vi "raster sequence build.vi"() -> ()   [LabVIEW 2017]
uses:
  Classes/Sequence/SequenceSubvis/TestStep-StepType.ctl
  Classes/Sequence/SequenceSubvis/TestStepTypes.ctl
  Classes/Sequence/SequenceSubvis/RF Direction.ctl
  Classes/Sequence/SequenceSubvis/PolarizationSelect.ctl
  Classes/aparCfg/rasterConfig.ctl
  Classes/VXMCfg/VXMCfg.lvclass
  Classes/aparCfg/aparCfg.lvclass
panel:
  out "size(s)":i32
  out "Total points":dbl
  out "Raster Sequence":T1[](array[typedef])
  in  "Polarization":enum16{"Vertical", "Horizontal", "Both"}(ring)=enum."Both"
  in  "RF In/Out":T3
  out "apar properties.RasterDef":T5={"Nyquist, mm"=28.0, "Window, cm"=42.0}
  in  "Cfg File path":path=path "C:/Users/Public/Documents/UCAR/APAR Board Test/SupportFiles/aparConfig.ini"
  in  "Motion64.ini path":path=path "C:/Users/Public/Documents/UCAR/APAR Board Test/SupportFiles/Motion64.ini"
  out "TestZT":cluster{"Z mm":dbl, "Horizontal T deg":dbl}={"Z mm"=0.0, "Horizontal T deg"=1.0}
  out "TestSequence for P&M":T1[](array[typedef])=[{"StepType"=enum."Motion", "RF In/Out"=enum."Tx - RF In", "Module/Raster"=0, "Polarization"=enum."Vertical", "PhaseShift deg"=[], "Attenuation dB"=[], "Position"={"X mm"=204.374756, "Y mm"=144.119598, "Z mm"=0.0, "T deg"=-89.0}, "Patch RF In/Out"=TRUE}, {"StepType"=enum."SweepTest", "RF In/Out"=enum."Tx - RF In", "Module/Raster"=0, "Polarization"=enum."Vertical", "PhaseShift deg"=[0.0, 5.625, 11.25], "Attenuation dB"=[0.0, 0.5], "Position"={"X mm"=0.0, "Y mm"=0.0, "Z mm"=0.0, "T deg"=0.0}, "Patch RF In/Out"=FALSE}, {"StepType"=enum."Motion", "RF In/Out"=enum."Tx - RF In", "Module/Raster"=0, "Polarization"=enum."Horizontal", "PhaseShift deg"=[], "Attenuation dB"=[], "Position"={"X mm"=204.374756, "Y mm"=144.119598, "Z mm"=0.0, "T deg"=1.0}, "Patch RF In/Out"=FALSE}, {"StepType"=enum."SweepTest", "RF In/Out"=enum."Tx - RF In", "Module/Raster"=0, "Polarization"=enum."Horizontal", "PhaseShift deg"=[0.0, 5.625, 11.25], "Attenuation dB"=[0.0, 0.5], "Position"={"X mm"=0.0, "Y mm"=0.0, "Z mm"=0.0, "T deg"=0.0}, "Patch RF In/Out"=FALSE}, {"StepType"=enum."Motion", "RF In/Out"=enum."Tx - RF In", "Module/Raster"=4, "Polarization"=enum."Vertical", "PhaseShift deg"=[], "Attenuation dB"=[], "Position"={"X mm"=315.230015, "Y mm"=144.76588, "Z mm"=0.0, "T deg"=-89.0}, "Patch RF In/Out"=FALSE}, {"StepType"=enum."SweepTest", "RF In/Out"=enum."Tx - RF In", "Module/Raster"=4, "Polarization"=enum."Vertical", "PhaseShift deg"=[0.0, 5.625, 11.25], "Attenuation dB"=[0.5], "Position"={"X mm"=0.0, "Y mm"=0.0, "Z mm"=0.0, "T deg"=0.0}, "Patch RF In/Out"=FALSE}, {"StepType"=enum."Motion", "RF In/Out"=enum."Tx - RF In", "Module/Raster"=4, "Polarization"=enum."Horizontal", "PhaseShift deg"=[], "Attenuation dB"=[], "Position"={"X mm"=315.230015, "Y mm"=144.76588, "Z mm"=0.0, "T deg"=1.0}, "Patch RF In/Out"=FALSE}, {"StepType"=enum."SweepTest", "RF In/Out"=enum."Tx - RF In", "Module/Raster"=4, "Polarization"=enum."Horizontal", "PhaseShift deg"=[0.0, 5.625, 11.25], "Attenuation dB"=[0.5], "Position"={"X mm"=0.0, "Y mm"=0.0, "Z mm"=0.0, "T deg"=0.0}, "Patch RF In/Out"=FALSE}, {"StepType"=enum."Motion", "RF In/Out"=enum."Tx - RF In", "Module/Raster"=7, "Polarization"=enum."Vertical", "PhaseShift deg"=[], "Attenuation dB"=[], "Position"={"X mm"=398.371459, "Y mm"=145.250591, "Z mm"=0.0, "T deg"=-89.0}, "Patch RF In/Out"=FALSE}, {"StepType"=enum."SweepTest", "RF In/Out"=enum."Tx - RF In", "Module/Raster"=7, "Polarization"=enum."Vertical", "PhaseShift deg"=[0.0], "Attenuation dB"=[0.0], "Position"={"X mm"=0.0, "Y mm"=0.0, "Z mm"=0.0, "T deg"=0.0}, "Patch RF In/Out"=FALSE}, {"StepType"=enum."Motion", "RF In/Out"=enum."Tx - RF In", "Module/Raster"=10, "Polarization"=enum."Vertical", "PhaseShift deg"=[], "Attenuation dB"=[], "Position"={"X mm"=259.640815, "Y mm"=172.156554, "Z mm"=0.0, "T deg"=-89.0}, "Patch RF In/Out"=FALSE}, {"StepType"=enum."SweepTest", "RF In/Out"=enum."Tx - RF In", "Module/Raster"=10, "Polarization"=enum."Vertical", "PhaseShift deg"=[22.5, 28.125], "Attenuation dB"=[6.0], "Position"={"X mm"=0.0, "Y mm"=0.0, "Z mm"=0.0, "T deg"=0.0}, "Patch RF In/Out"=FALSE}, {"StepType"=enum."Motion", "RF In/Out"=enum."Tx - RF In", "Module/Raster"=10, "Polarization"=enum."Horizontal", "PhaseShift deg"=[], "Attenuation dB"=[], "Position"={"X mm"=259.640815, "Y mm"=172.156554, "Z mm"=0.0, "T deg"=1.0}, "Patch RF In/Out"=FALSE}, {"StepType"=enum."SweepTest", "RF In/Out"=enum."Tx - RF In", "Module/Raster"=10, "Polarization"=enum."Horizontal", "PhaseShift deg"=[22.5, 28.125], "Attenuation dB"=[6.0], "Position"={"X mm"=0.0, "Y mm"=0.0, "Z mm"=0.0, "T deg"=0.0}, "Patch RF In/Out"=FALSE}, {"StepType"=enum."Motion", "RF In/Out"=enum."Tx - RF In", "Module/Raster"=13, "Polarization"=enum."Vertical", "PhaseShift deg"=[], "Attenuation dB"=[], "Position"={"X mm"=342.782259, "Y mm"=172.641265, "Z mm"=0.0, "T deg"=-89.0}, "Patch RF In/Out"=FALSE}, {"StepType"=enum."SweepTest", "RF In/Out"=enum."Tx - RF In", "Module/Raster"=13, "Polarization"=enum."Vertical", "PhaseShift deg"=[45.0], "Attenuation dB"=[0.0], "Position"={"X mm"=0.0, "Y mm"=0.0, "Z mm"=0.0, "T deg"=0.0}, "Patch RF In/Out"=FALSE}, {"StepType"=enum."Motion", "RF In/Out"=enum."Tx - RF In", "Module/Raster"=15, "Polarization"=enum."Vertical", "PhaseShift deg"=[], "Attenuation dB"=[], "Position"={"X mm"=398.209889, "Y mm"=172.964406, "Z mm"=0.0, "T deg"=-89.0}, "Patch RF In/Out"=FALSE}, {"StepType"=enum."SweepTest", "RF In/Out"=enum."Tx - RF In", "Module/Raster"=15, "Polarization"=enum."Vertical", "PhaseShift deg"=[0.0], "Attenuation dB"=[0.0], "Position"={"X mm"=0.0, "Y mm"=0.0, "Z mm"=0.0, "T deg"=0.0}, "Patch RF In/Out"=FALSE}, {"StepType"=enum."Motion", "RF In/Out"=enum."Rx - RF Out", "Module/Raster"=4, "Polarization"=enum."Vertical", "PhaseShift deg"=[], "Attenuation dB"=[], "Position"={"X mm"=315.230015, "Y mm"=144.76588, "Z mm"=0.0, "T deg"=-89.0}, "Patch RF In/Out"=TRUE}, {"StepType"=enum."SweepTest", "RF In/Out"=enum."Rx - RF Out", "Module/Raster"=4, "Polarization"=enum."Vertical", "PhaseShift deg"=[0.0, 5.625, 11.25], "Attenuation dB"=[0.5], "Position"={"X mm"=0.0, "Y mm"=0.0, "Z mm"=0.0, "T deg"=0.0}, "Patch RF In/Out"=FALSE}, {"StepType"=enum."Motion", "RF In/Out"=enum."Rx - RF Out", "Module/Raster"=4, "Polarization"=enum."Horizontal", "PhaseShift deg"=[], "Attenuation dB"=[], "Position"={"X mm"=315.230015, "Y mm"=144.76588, "Z mm"=0.0, "T deg"=1.0}, "Patch RF In/Out"=FALSE}, {"StepType"=enum."SweepTest", "RF In/Out"=enum."Rx - RF Out", "Module/Raster"=4, "Polarization"=enum."Horizontal", "PhaseShift deg"=[0.0, 5.625, 11.25], "Attenuation dB"=[0.5], "Position"={"X mm"=0.0, "Y mm"=0.0, "Z mm"=0.0, "T deg"=0.0}, "Patch RF In/Out"=FALSE}, {"StepType"=enum."Motion", "RF In/Out"=enum."Rx - RF Out", "Module/Raster"=12, "Polarization"=enum."Vertical", "PhaseShift deg"=[], "Attenuation dB"=[], "Position"={"X mm"=315.068444, "Y mm"=172.479695, "Z mm"=0.0, "T deg"=-89.0}, "Patch RF In/Out"=FALSE}, {"StepType"=enum."SweepTest", "RF In/Out"=enum."Rx - RF Out", "Module/Raster"=12, "Polarization"=enum."Vertical", "PhaseShift deg"=[0.0, 5.625, 11.25], "Attenuation dB"=[0.0, 0.5], "Position"={"X mm"=0.0, "Y mm"=0.0, "Z mm"=0.0, "T deg"=0.0}, "Patch RF In/Out"=FALSE}, {"StepType"=enum."Motion", "RF In/Out"=enum."Rx - RF Out", "Module/Raster"=12, "Polarization"=enum."Horizontal", "PhaseShift deg"=[], "Attenuation dB"=[], "Position"={"X mm"=315.068444, "Y mm"=172.479695, "Z mm"=0.0, "T deg"=1.0}, "Patch RF In/Out"=FALSE}, {"StepType"=enum."SweepTest", "RF In/Out"=enum."Rx - RF Out", "Module/Raster"=12, "Polarization"=enum."Horizontal", "PhaseShift deg"=[0.0, 5.625, 11.25], "Attenuation dB"=[0.0, 0.5], "Position"={"X mm"=0.0, "Y mm"=0.0, "Z mm"=0.0, "T deg"=0.0}, "Patch RF In/Out"=FALSE}, {"StepType"=enum."Finish", "RF In/Out"=enum."Tx - RF In", "Module/Raster"=0, "Polarization"=enum."Vertical", "PhaseShift deg"=[], "Attenuation dB"=[], "Position"={"X mm"=0.0, "Y mm"=0.0, "Z mm"=0.0, "T deg"=0.0}, "Patch RF In/Out"=FALSE}]
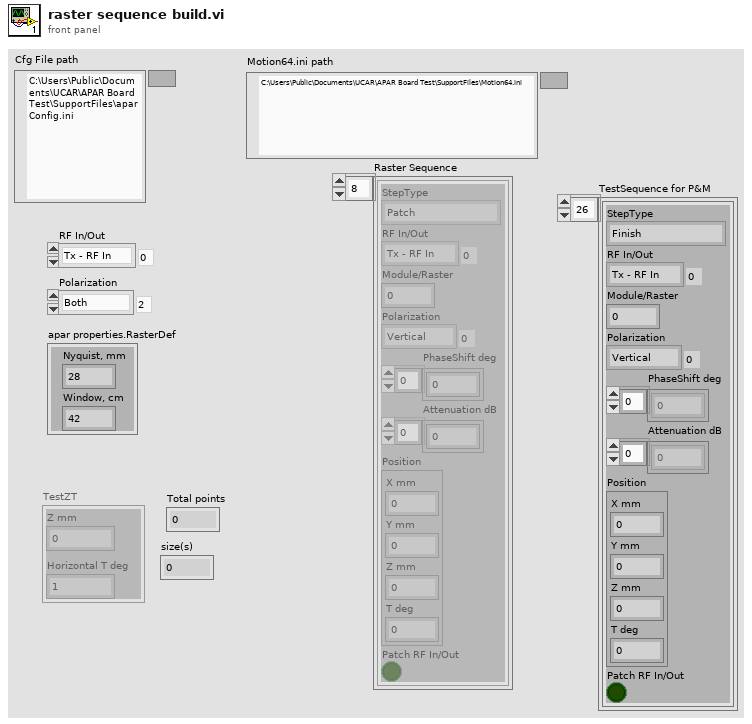
[diagram p1: front panel]
types:
  T1 = typedef "TestStep-StepType.ctl" = cluster{"StepType":T2, "RF In/Out":T3, "Module/Raster":i32, "Polarization":T4, "PhaseShift deg":dbl[], "Attenuation dB":dbl[], "Position":cluster{"X mm":dbl, "Y mm":dbl, "Z mm":dbl, "T deg":dbl}, "Patch RF In/Out":bool}
  T2 = typedef "TestStepTypes.ctl" = enum16{"Patch", "Motion", "SweepTest", "RasterTest", "Finish"}
  T3 = typedef "RF Direction.ctl" = enum16{"Tx - RF In", "Rx - RF Out"}
  T4 = typedef "PolarizationSelect.ctl" = enum16{"Vertical", "Horizontal"}
  T5 = typedef "rasterConfig.ctl" = cluster{"Nyquist, mm":dbl, "Window, cm":dbl}
  T6 = cluster{"X step":dbl, "Y step":dbl, "Z step":dbl, "T step":dbl}[]
  T7 = cluster{"X mm":dbl, "Y mm":dbl, "Z mm":dbl, "T deg.":dbl}[]
  T8 = cluster{"X mm":dbl, "Y mm":dbl, "Z mm":dbl, "T deg":dbl}
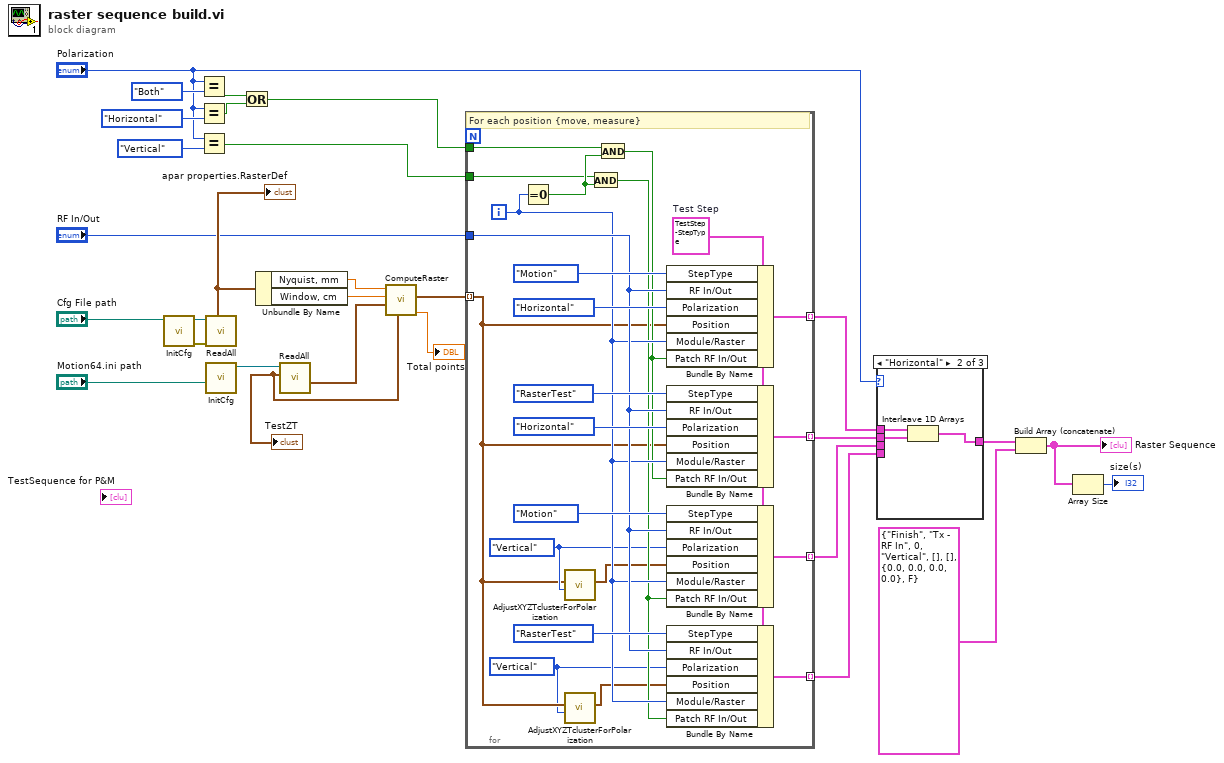
[diagram p0: block diagram]
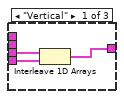
[diagram p2: hidden frame]
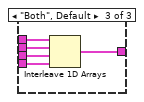
[diagram p3: hidden frame]
diagram:
  n1 = call "InitCfg.vi"("Cfg File path"="Cfg File path") -> ("error out"=w27:errorcluster, "aparCfg out"=w26:refnum<class "aparCfg.lvclass">)  [unwired: 9 in]
  n2 = Equal?(x="Polarization", y=enum16{"Vertical", "Horizontal", "Both"}."Both" ("Polarization")) -> (x = y?=w7:bool)
  n3 = Equal?(x="Polarization", y=enum16{"Vertical", "Horizontal", "Both"}."Horizontal" ("Polarization")) -> (x = y?=w6:bool)
  n4 = Equal?(x="Polarization", y=enum16{"Vertical", "Horizontal", "Both"}."Vertical" ("Polarization")) -> (x = y?=w4:bool)
  n5 = call "ReadAll.vi"("error in (no error)"=w27, "aparCfg in"=w26) -> ("apar properties.RasterDef"=w24:T5)  [unwired: 2 in, 7 out]
  "apar properties.RasterDef" <- w24
  n6 = call "InitCfg.vi"("Cfg File path"="Motion64.ini path") -> ("VXMCfg out"=w28:refnum<class "VXMCfg.lvclass">)  [unwired: 9 in, 1 out]
  n7 = Or(x=w7, y=w6) -> (x .or. y?=w5:bool)
  n8 = Unbundle By Name(w24) -> ("Nyquist, mm"=w23:dbl, "Window, cm"=w22:dbl)
  n9 = call "ReadAll.vi"("VXMCfg in"=w28) -> ("Position Array"=w21:T6, "TestZT"=w18:cluster{"Z mm":dbl, "Horizontal T deg":dbl})  [unwired: 1 in, 8 out]
  "TestZT" <- w18
  n10 = call "ComputeRaster.vi"("TestZT"=w18, "Position Array in"=w21, "Window dimension"=w22, "Nyquist, mm"=w23) -> ("Total points"=→"Total points":dbl, "Position Array out"=w20:T7)  [unwired: 4 in, 2 out]
  n11 = for {
    tunnel: w20 -> [w32] mode=indexing
    tunnel: "RF In/Out" -> [w44]
    tunnel: [w48] -> w17 mode=indexing
    tunnel: [w47] -> w16 mode=indexing
    tunnel: [w42] -> w14 mode=indexing
    tunnel: [w41] -> w13 mode=indexing
    tunnel: w5 -> [w37]
    tunnel: w4 -> [w36]
    i -> [w40]
    w31 = PolarizationSelect."Vertical" ("Polarization")
    w33 = PolarizationSelect."Vertical" ("Polarization")
    w43 = T1 {"StepType"=enum."Motion", "RF In/Out"=enum."Tx - RF In", "Module/Raster"=0, "Polarization"=enum."Horizontal", "PhaseShift deg"=[], "Attenuation dB"=[], "Position"={"X mm"=0.0, "Y mm"=0.0, "Z mm"=0.0, "T deg"=0.0}, "Patch RF In/Out"=FALSE}  # Test Step
    # "For each position {move, measure}"
    n12 = Equal To 0?(x=w40) -> (x = 0?=w39:bool)
    n13 = call "AdjustXYZTclusterForPolarization.vi"("Polarization"=w33, "Position, Horizontal"=w32) -> ("Position out"=w34:T8)  [unwired: 9 in]
    n14 = call "AdjustXYZTclusterForPolarization.vi"("Polarization"=w31, "Position, Horizontal"=w32) -> ("Position out"=w30:T8)  [unwired: 9 in]
    n15 = And(x=w36, y=w39) -> (x .and. y?=w35:bool)
    n16 = And(x=w37, y=w39) -> (x .and. y?=w38:bool)
    n17 = Bundle By Name(cluster=w43, "StepType"=TestStepTypes."Motion", "RF In/Out"=w44, "Polarization"=PolarizationSelect."Horizontal", "Position"=w32, "Module/Raster"=w40, "Patch RF In/Out"=w38) -> (w48:T1)
    n18 = Bundle By Name(cluster=w43, "StepType"=TestStepTypes."RasterTest", "RF In/Out"=w44, "Polarization"=PolarizationSelect."Horizontal", "Position"=w32, "Module/Raster"=w40, "Patch RF In/Out"=w38) -> (w47:T1)
    n19 = Bundle By Name(cluster=w43, "StepType"=TestStepTypes."Motion", "RF In/Out"=w44, "Polarization"=w33, "Position"=w34, "Module/Raster"=w40, "Patch RF In/Out"=w35) -> (w42:T1)
    n20 = Bundle By Name(cluster=w43, "StepType"=TestStepTypes."RasterTest", "RF In/Out"=w44, "Polarization"=w31, "Position"=w30, "Module/Raster"=w40, "Patch RF In/Out"=w35) -> (w41:T1)
  }
  n21 = case shown="\"Horizontal\"" "Polarization" {
    tunnel: w17 -> [_ w58 w63]
    tunnel: w16 -> [_ w57 w62]
    tunnel: w14 -> [w55 _ w61]
    tunnel: w13 -> [w54 _ w60]
    tunnel: [w53 w56 w59] -> w12
    frame "Vertical" {
      n22 = Interleave 1D Arrays(w55, w54) -> (w53:T1[])
    }
    frame "Horizontal" {
      n23 = Interleave 1D Arrays(w58, w57) -> (w56:T1[])
    }
    frame "Both", Default {
      n24 = Interleave 1D Arrays(w63, w62, w61, w60) -> (w59:T1[])
    }
  }
  n25 = Build Array (concatenate)(w12, T1 {"StepType"=enum."Finish", "RF In/Out"=enum."Tx - RF In", "Module/Raster"=0, "Polarization"=enum."Vertical", "PhaseShift deg"=[], "Attenuation dB"=[], "Position"={"X mm"=0.0, "Y mm"=0.0, "Z mm"=0.0, "T deg"=0.0}, "Patch RF In/Out"=FALSE} ("Test")) -> (w2:T1[])
  "Raster Sequence" <- w2
  n26 = Array Size(array=w2) -> (size(s)=→"size(s)":i32)
